vi "To and  From String Array.vi"() -> (0 "error out":errorcluster, 3 "Pass":bool)   [LabVIEW 2014, in "DAQmx Module Tests.lvlib"]
uses:
  DAQmx Module Tests.lvlib
  <vilib>/NI/Tag Bus Module Framework/channel/channel classification.ctl
  <vilib>/NI/Tag Bus/tag/Data Type.ctl
  module/configuration/DAQmx Module Configuration.lvclass/DAQmx Module Configuration.ctl
  <vilib>/NI/Tag Bus Module Framework/channel/TBM channel.lvclass/TBM channel.ctl
  <vilib>/NI/Tag Bus/tag/tag descriptor.lvclass/tag descriptor.ctl
  <vilib>/NI/Tag Bus Module Framework/channel/TBM channel.lvclass
  module/configuration/DAQmx Module Configuration.lvclass
  <vilib>/NI/Tag Bus/tag/tag descriptor.lvclass
panel:
  out "data type 2":T1
  out "data type":T1
  in  "index":i32
  out "name 2":string
  out "name":string
  out "channel classification 2":T2
  out "channel classification":T2
  out "x = y?":T3(array[cluster])
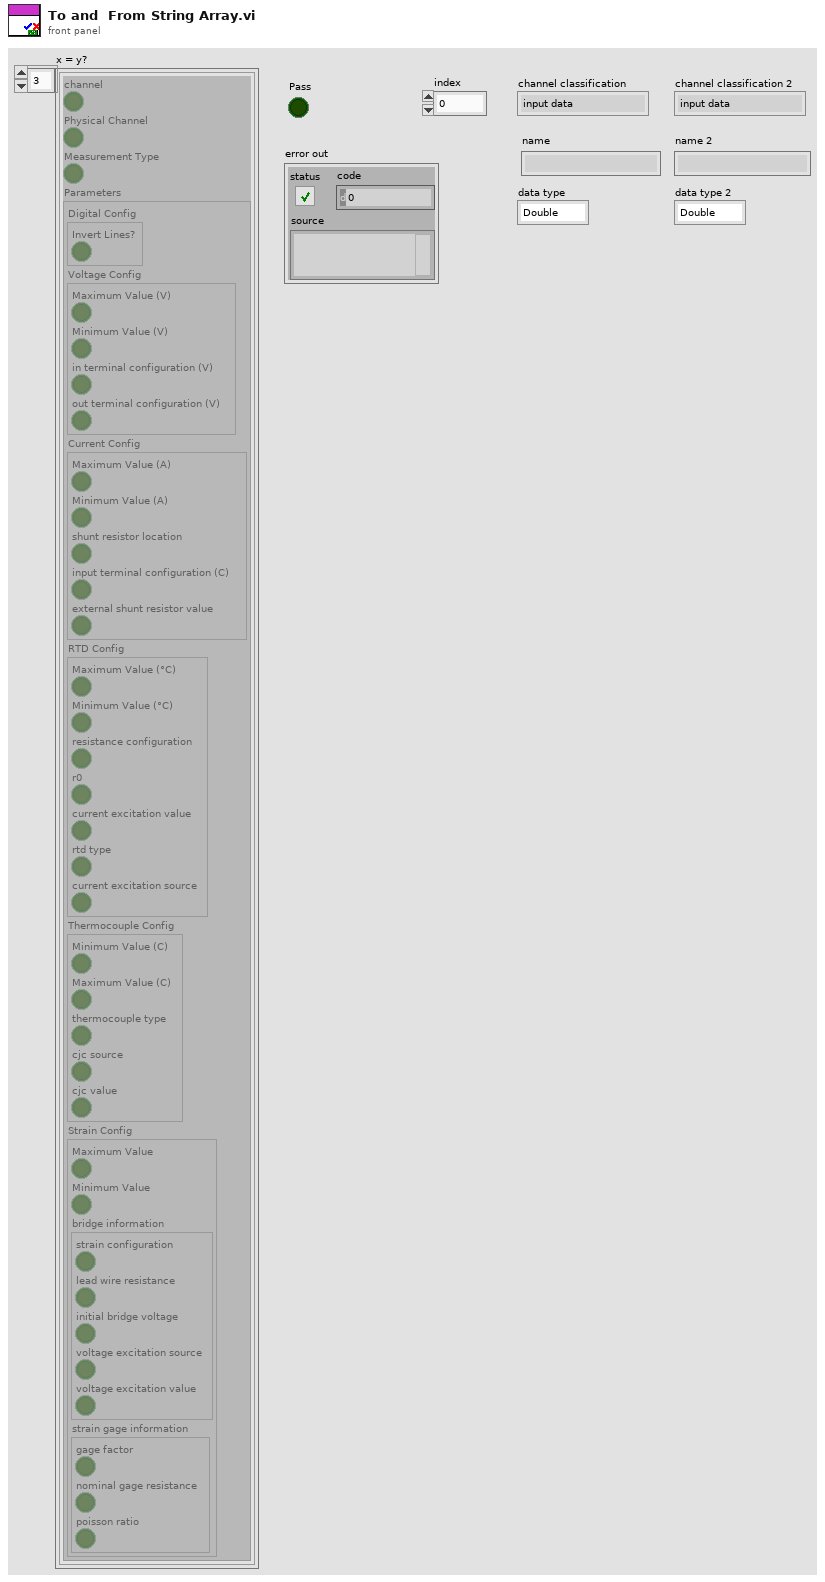
[diagram p1: front panel]
types:
  T1 = typedef "tag bus.lvlib/tag descriptor.lvclass/Data Type.ctl" = enum16{"Double", "Single", "I64", "I32", "I16", "I8", "U64", "U32", "U16", "U8", "Boolean", "String", "Array of Double", "Array of Single", "Array of I64", "Array of I32", "Array of I16", "Array of I8", "Array of U64", "Array of U32", "Array of U16", "Array of U8", "Array of Boolean", "Array of String"}
  T2 = typedef "TBM channel.lvclass/channel classification.ctl" = enum16{"input data", "output data", "processing parameter", "processing result"}
  T3 = cluster{"channel":bool, "Physical Channel":bool, "Measurement Type":bool, "Parameters":cluster{"Digital Config":cluster{"Invert Lines?":bool}, "Voltage Config":cluster{"Maximum Value (V)":bool, "Minimum Value (V)":bool, "in terminal configuration (V)":bool, "out terminal configuration (V)":bool}, "Current Config":cluster{"Maximum Value (A)":bool, "Minimum Value (A)":bool, "shunt resistor location":bool, "input terminal configuration (C)":bool, "external shunt resistor value":bool}, "RTD Config":cluster{"Maximum Value (°C)":bool, "Minimum Value (°C)":bool, "resistance configuration":bool, "r0":bool, "current excitation value":bool, "rtd type":bool, "current excitation source":bool}, "Thermocouple Config":cluster{"Minimum Value (C)":bool, "Maximum Value (C)":bool, "thermocouple type":bool, "cjc source":bool, "cjc value":bool}, "Strain Config":cluster{"Maximum Value":bool, "Minimum Value":bool, "bridge information":cluster{"strain configuration":bool, "lead wire resistance":bool, "initial bridge voltage":bool, "voltage excitation source":bool, "voltage excitation value":bool}, "strain gage information":cluster{"gage factor":bool, "nominal gage resistance":bool, "poisson ratio":bool}}}}[]
  T4 = typedef "DAQmx Module Configuration.lvclass/Line.ctl" = cluster{"channel":refnum<class "TBM channel.lvclass">, "Physical Channel":string, "Measurement Type":T5, "Parameters":T6}
  T5 = typedef "DAQmx Module Configuration.lvclass/Measurement Type.ctl" = enum16{"Digital Input", "Digital Output", "Voltage Input", "Voltage Output", "Current Input", "Current Output", "RTD", "Thermocouple", "Strain"}
  T6 = typedef "DAQmx Module Configuration.lvclass/Parameters.ctl" = cluster{"Digital Config":cluster{"Invert Lines?":bool}, "Voltage Config":cluster{"Maximum Value (V)":dbl, "Minimum Value (V)":dbl, "in terminal configuration (V)":i32, "out terminal configuration (V)":i32}, "Current Config":cluster{"Maximum Value (A)":dbl, "Minimum Value (A)":dbl, "shunt resistor location":i32, "input terminal configuration (C)":i32, "external shunt resistor value":dbl}, "RTD Config":cluster{"Maximum Value (°C)":dbl, "Minimum Value (°C)":dbl, "resistance configuration":i32, "r0":dbl, "current excitation value":dbl, "rtd type":i32, "current excitation source":i32}, "Thermocouple Config":cluster{"Minimum Value (C)":dbl, "Maximum Value (C)":dbl, "thermocouple type":i32, "cjc source":i32, "cjc value":dbl}, "Strain Config":cluster{"Maximum Value":dbl, "Minimum Value":dbl, "bridge information":cluster{"strain configuration":i32, "lead wire resistance":dbl, "initial bridge voltage":dbl, "voltage excitation source":i32, "voltage excitation value":dbl}, "strain gage information":cluster{"gage factor":dbl, "nominal gage resistance":dbl, "poisson ratio":dbl}}}
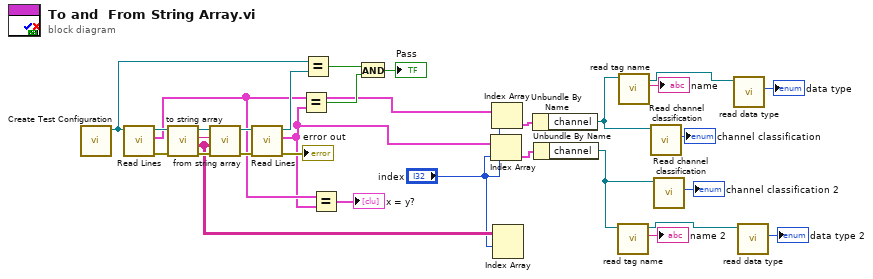
[diagram p0: block diagram]
diagram:
  n1 = call "Create Test Configuration.vi"() -> ("Module Configuration"=w22:refnum<class "DAQmx Module Configuration.lvclass">)  [unwired: 6 in, 5 out]
  n2 = call "Read Lines.vi"("Daqmx Module configuration in"=w22) -> ("error out"=w26:errorcluster, "Lines"=w16:T4[], "Daqmx Module configuration out"=w28:refnum<class "DAQmx Module Configuration.lvclass">)  [unwired: 8 in]
  n3 = call-dynamic "to string array.vi"("error in (no error)"=w26, "module configuration in"=w28) -> ("error out"=w25:errorcluster, "Array"=w2:string[][], "version"=w30:string, "module configuration out"=w29:refnum<class "DAQmx Module Configuration.lvclass">)  [unwired: 6 in]
  n4 = call-dynamic "from string array.vi"("error in (no error)"=w25, "String Array"=w2, "version"=w30, "module configuration in"=w29) -> ("error out"=w24:errorcluster, "module configuration out"=w27:refnum<class "DAQmx Module Configuration.lvclass">)  [unwired: 6 in]
  n5 = call "Read Lines.vi"("error in (no error)"=w24, "Daqmx Module configuration in"=w27) -> ("error out"=→"error out":errorcluster, "Lines"=w15:T4[], "Daqmx Module configuration out"=w21:refnum<class "DAQmx Module Configuration.lvclass">)  [unwired: 7 in]
  n6 = Equal?(x=w16, y=w15) -> (x = y?=w19:bool)
  n7 = Equal?(x=w22, y=w21) -> (x = y?=w20:bool)
  n8 = Equal?(x=w16, y=w15) -> (x = y?=→"x = y?":T3)
  n9 = And(x=w20, y=w19) -> (x .and. y?=→"Pass":bool)
  n10 = Index Array(array=w15, index="index") -> (element=w13:T4)
  n11 = Index Array(array=w16, index="index") -> (element=w14:T4)
  n12 = Index Array(array=w2, index (row)="index") -> ()  [unwired: 1 in, 1 out]
  n13 = Unbundle By Name(w14) -> ("channel"=w10:refnum<class "TBM channel.lvclass">)
  n14 = Unbundle By Name(w13) -> ("channel"=w9:refnum<class "TBM channel.lvclass">)
  n15 = call <vilib>:"read tag name.vi"("system tag in"=w9) -> ("name"=→"name 2":string, "system tag out"=w5:refnum<class "TBM channel.lvclass">)  [unwired: 8 in, 1 out]
  n16 = call <vilib>:"read tag name.vi"("system tag in"=w10) -> ("name"=→"name":string, "system tag out"=w6:refnum<class "TBM channel.lvclass">)  [unwired: 8 in, 1 out]
  n17 = call <vilib>:"Read channel classification.vi"("channel in"=w10) -> ("channel classification"=→"channel classification":T2)  [unwired: 8 in, 2 out]
  n18 = call <vilib>:"Read channel classification.vi"("channel in"=w9) -> ("channel classification"=→"channel classification 2":T2)  [unwired: 8 in, 2 out]
  n19 = call <vilib>:"read data type.vi"("system tag in"=w6) -> ("data type"=→"data type":T1)  [unwired: 8 in, 2 out]
  n20 = call <vilib>:"read data type.vi"("system tag in"=w5) -> ("data type"=→"data type 2":T1)  [unwired: 8 in, 2 out]
